vi "Fit.vi"(8 "error in (no error)":errorcluster caption="entrée d'erreur (pas d'erreur)", 9 "y":string[][](array[string]), 10 "X":string[][](array[string]), 11 "KBinsDiscretizer.lvclass":refnum<class "KBinsDiscretizer.lvclass">) -> (0 "error out":errorcluster caption="sortie d'erreur", 2 "String Data":string, 3 "KBinsDiscretizer.lvclass":refnum<class "KBinsDiscretizer.lvclass">)   [LabVIEW 2020, in "KBinsDiscretizer.lvclass"]
doc: "Fit the estimator.\n\nReturns : \n\n- String : OK"
uses:
  KBinsDiscretizer.lvclass
  KBinsDiscretizer.lvclass/KBinsDiscretizer.ctl
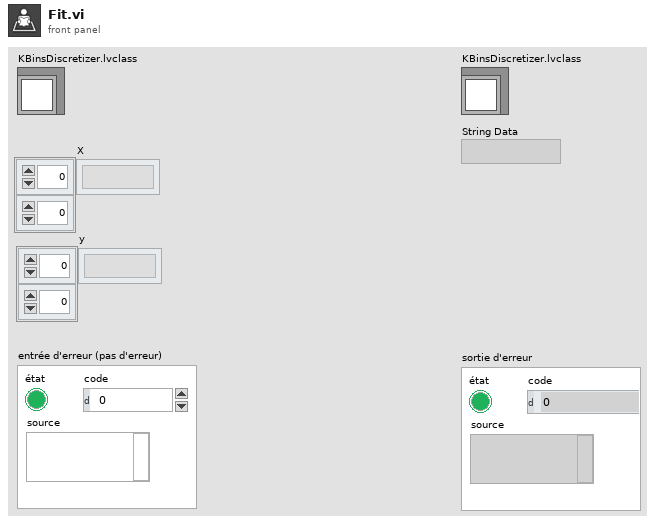
[diagram p1: front panel]
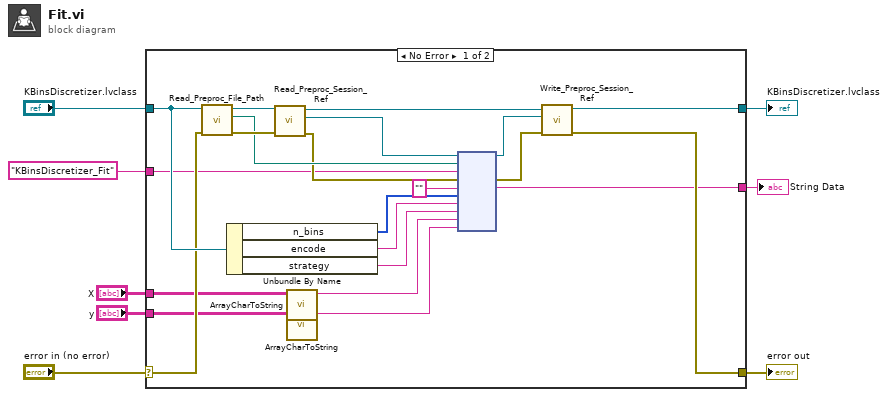
[diagram p0: block diagram]
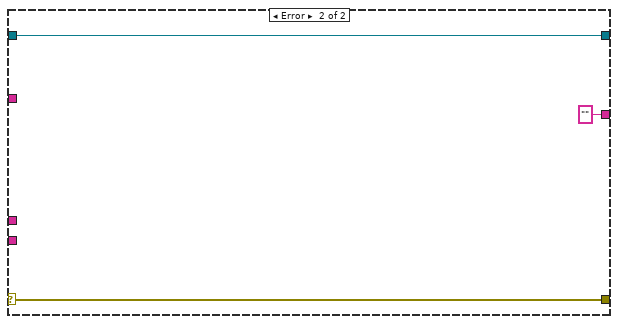
[diagram p2: hidden frame]
diagram:
  n1 = case shown="No Error" "error in (no error)" {
    selector: "error in (no error)" -> [w20 w33]
    tunnel: [w19 w33] -> w7
    tunnel: [w13 w32] -> w5
    tunnel: "KBinsDiscretizer.lvclass" -> [w21 w32]
    tunnel: "KBinsDiscretizer_Fit" ("Fonction") -> [w15 _]
    tunnel: [w14 ""] -> w3
    tunnel: "X" -> [w12 _]
    tunnel: "y" -> [w11 _]
    frame No Error {
      n2 = call-dynamic "Read_Preproc_File_Path.vi"("error in (no error)"=w20, "Python in"=w21) -> ("error out"=w29:errorcluster, "File_Path"=w26:path, "Python out"=w30:refnum<class "KBinsDiscretizer.lvclass">)  [unwired: 7 in]
      n3 = Unbundle By Name(w21) -> ("n_bins"=w18:i32[], "encode"=w17:string, "strategy"=w16:string)
      n4 = call-dynamic "Read_Preproc_Session_Ref.vi"("error in (no error)"=w29, "Python in"=w30) -> ("error out"=w25:errorcluster, "Session_ref"=w27:refnum<k35>, "Python out"=w28:refnum<class "KBinsDiscretizer.lvclass">)  [unwired: 7 in]
      n5 = call "ArrayCharToString.vi"("TAB"=w12) -> ("Instruction"=w10:string)  [unwired: 10 in]
      n6 = call "ArrayCharToString.vi"("TAB"=w11) -> ("Instruction"=w9:string)  [unwired: 10 in]
      n7 = node(w27, w26, w15, w25, "", w18, w17, w16, w10, w9) -> (w23:refnum<k35>, w24:errorcluster, w14:string)  [unwired: 5 in, 2 out]
      n8 = call-dynamic "Write_Preproc_Session_Ref.vi"("error in (no error)"=w24, "Session_ref"=w23, "Python in"=w28) -> ("error out"=w19:errorcluster, "Python out"=w13:refnum<class "KBinsDiscretizer.lvclass">)  [unwired: 7 in]
    }
    frame Error {
    }
  }
  "error out" <- w7
  "KBinsDiscretizer.lvclass" <- w5
  "String Data" <- w3
